vi "Wait for Registrations.vi"(8 "error in":errorcluster, 9 "Wait for Reg Confirmation? (F)":bool, 10 "Timeout (5 sec)":i32=5000, 11 "Module Data In":refnum<class "Rename.lvclass">) -> (0 "error out":errorcluster, 2 "timed out?":bool, 3 "Module Data Out":refnum<class "Rename.lvclass">)   [LabVIEW 2015, in "Generic Module Library.lvlib" / "Template G_Module.lvlib"]
uses:
  Template G_Module.lvlib
  Module Broadcasts/Broadcast Support/Registration Actions.ctl
  Module Class/Rename.lvclass
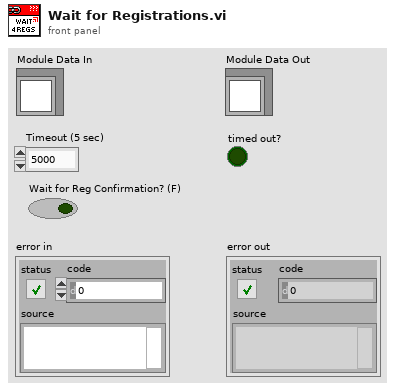
[diagram p1: front panel]
types:
  T1 = typedef "Generic Module Library.lvlib/Template G_Module.lvlib/Registration Actions.ctl" = enum16{"Create", "Get", "Destroy"}
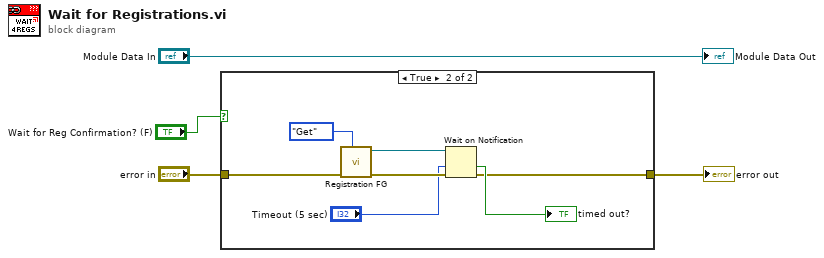
[diagram p0: block diagram]
diagram:
  n1 = case shown="True" "Wait for Reg Confirmation? (F)" {
    tunnel: "error in" -> [w5 w12]
    tunnel: [w5 w6] -> w1
    frame False {
    }
    frame True {
      n2 = call "Registration FG.vi"("Registration Actions"=Registration_Actions."Get", "error in"=w12) -> ("error out"=w11:errorcluster, "notifier out"=w9:refnum<notifier>)  [unwired: 8 in]
      n3 = Wait on Notification(notifier=w9, timeout in ms (-1)="Timeout (5 sec)", error in (no error)=w11) -> (timed out?=→"timed out?":bool, error out=w6:errorcluster)  [unwired: 1 in, 2 out]
    }
  }
  "error out" <- w1
  "Module Data Out" <- "Module Data In"
